vi "GetPersistentConfiguration.vi"(8 "Error In":errorcluster, 9 "DataIn":variant, 11 "reference in":refnum<class "UserManager.lvclass">) -> (0 "Error Out":errorcluster, 1 "DataOut":variant, 3 "reference out":refnum<class "UserManager.lvclass">)   [LabVIEW 2021, in "UserMananger.lvlib" / "UserManager.lvclass"]
uses:
  UserManager.lvclass
  Library_TAF_ApplicationFramework/TAFBaseGUI/TAFBaseGUI.lvclass
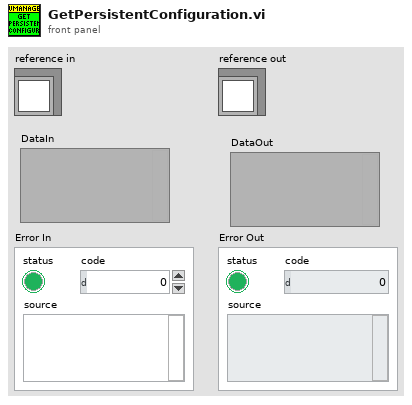
[diagram p1: front panel]
types:
  T1 = typedef "UserMananger.lvlib/UserManager.lvclass/ObjectAttributes.ctl" = cluster{"Interfaces":cluster{"ActivationUpdated":refnum<class "IAuthorizationUpdated.lvclass">}, "Locals":cluster{"MainGUIActive":refnum<queue>, "Evaluations":cluster{"Label":string, "Value":string}[]}, "Persistent":cluster{"Dummy":bool}}
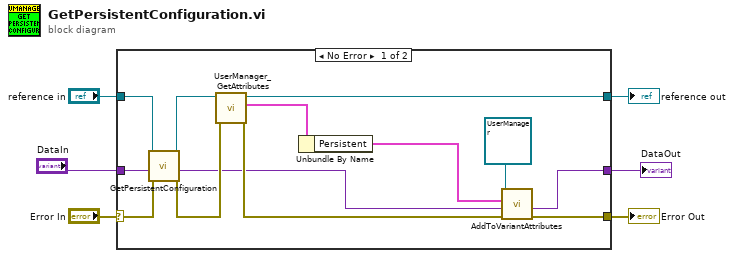
[diagram p0: block diagram]
diagram:
  n1 = case shown="No Error" "Error In" {
    selector: "Error In" -> [w19 w22]
    tunnel: [w16 w22] -> w5
    tunnel: [w15 w21] -> w3
    tunnel: "reference in" -> [w10 w21]
    tunnel: [w14 w20] -> w2
    tunnel: "DataIn" -> [w8 w20]
    frame No Error {
      n2 = call-parent "GetPersistentConfiguration.vi"("Error In"=w19, "DataIn"=w8, "reference in"=w10) -> ("Error Out"=w11:errorcluster, "DataOut"=w7:variant, "reference out"=w9:refnum<class "UserManager.lvclass">)  [unwired: 6 in]
      n3 = call "UserManager_GetAttributes.vi"("error in (no error)"=w11, "reference in"=w9) -> ("error out"=w17:errorcluster, "Data"=w18:T1, "reference out"=w15:refnum<class "UserManager.lvclass">)  [unwired: 6 in, 1 out]
      n4 = Unbundle By Name(w18) -> ("Persistent"=w13:cluster{"Dummy":bool})
      n5 = call "AddToVariantAttributes.vi"("error in (no error)"=w17, "DataIn in"=w7, "PersistentData"=w13, "Object"=refnum<class "UserManager.lvclass"> refnum ("VerticalButtonBar")) -> ("error out"=w16:errorcluster, "DataIn out"=w14:variant)  [unwired: 6 in]
    }
    frame Error {
    }
  }
  "Error Out" <- w5
  "reference out" <- w3
  "DataOut" <- w2
